vi "Get Data and Series JSON Settings.vi"(6 "Value Only":bool, 8 "error in (no error)":errorcluster, 9 "Width":u32, 10 "XY Data":variant, 11 "XYGraph in":refnum<vi>) -> (0 "error out":errorcluster, 1 "Minimums":dbl[](array[numeric]), 2 "Maximums":dbl[](array[numeric]), 3 "Series JSON":string, 4 "Plot Y Scale Index":u32[](array[numeric]), 5 "Data JSON":string)   [LabVIEW 2015, in "Front Panel Publisher.lvlib" / "Graph.lvclass"]
uses:
  Graph.lvclass
  <vilib>/Analysis/1siggen.llb/Ramp Pattern by Samples.vi
  <vilib>/gmath/NI_Gmath.lvlib
  <vilib>/Analysis/NI_AALBase.lvlib
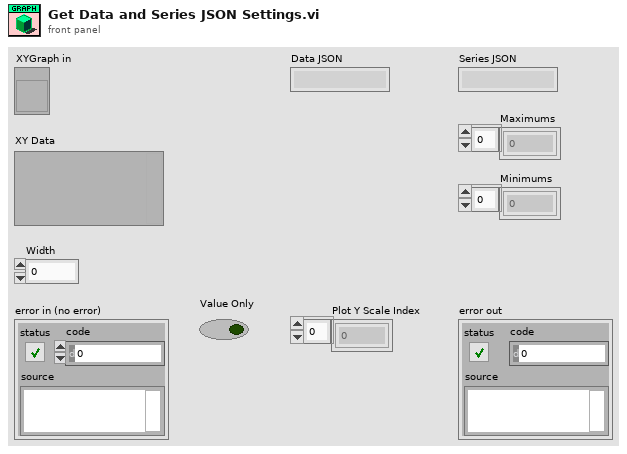
[diagram p1: front panel]
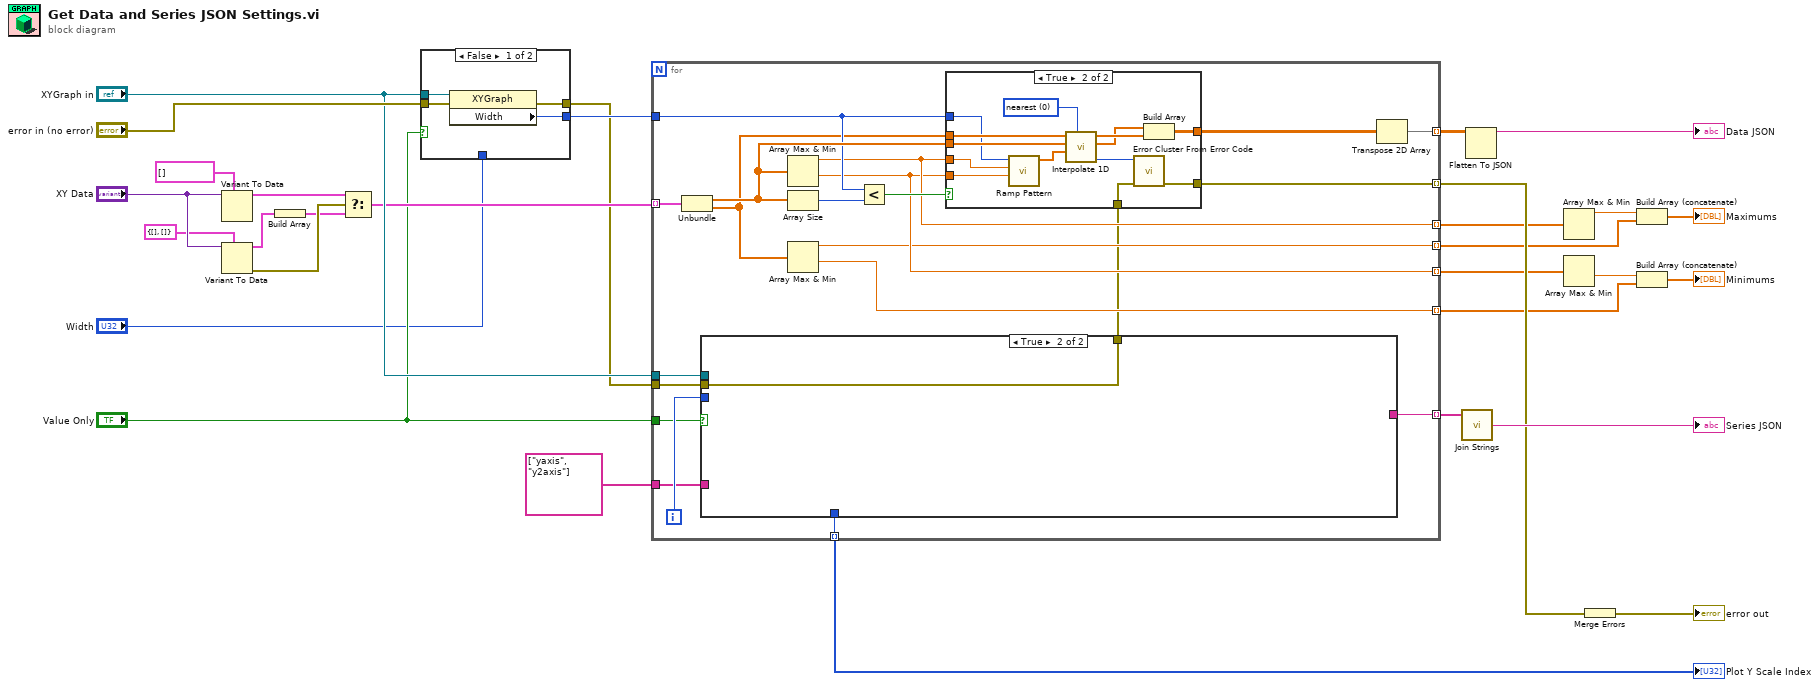
[diagram p0: block diagram]
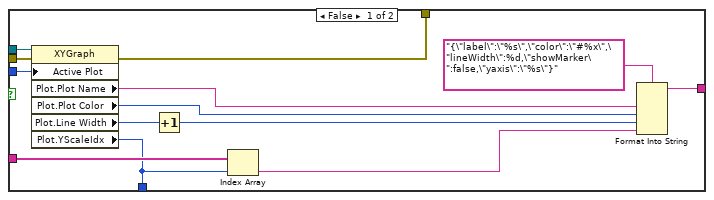
[diagram p3: hidden frame]
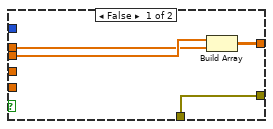
[diagram p4: hidden frame]
diagram:
  n1 = Variant To Data(type=cluster{dbl[], dbl[]}[] [], Variant="XY Data") -> (data=w15:cluster{dbl[], dbl[]}[])  [unwired: 1 in, 1 out]
  n2 = Variant To Data(type=cluster{dbl[], dbl[]} {[], []}, Variant="XY Data") -> (data=w14:cluster{dbl[], dbl[]}, error out=w16:errorcluster)  [unwired: 1 in]
  n3 = Build Array(w14) -> (w13:cluster{dbl[], dbl[]}[])
  n4 = Select(t=w15, s=w16, f=w13) -> (s? t:f=w12:cluster{dbl[], dbl[]}[])
  n5 = case shown="False" "Value Only" {
    tunnel: "error in (no error)" -> [w34 w36]
    tunnel: [w33 w35] -> w26
    tunnel: "XYGraph in" -> [w32 _]
    tunnel: [w31 w36] -> w3
    tunnel: "Width" -> [_ w35]
    frame False {
      n6 = property class="XYGraph"(reference=w32, error in=w34) -> (error out=w31:errorcluster, "Width"=w33:u32)  [unwired: 1 out]
    }
    frame True {
    }
  }
  n7 = for {
    tunnel: [w56] -> w24 mode=indexing
    tunnel: w12 -> [w54] mode=indexing
    tunnel: "XYGraph in" -> [w47]
    tunnel: [w57] -> w21 mode=indexing
    tunnel: w26 -> [w50]
    tunnel: string[] ["yaxis", "y2axis"] -> [w48]
    tunnel: [w46] -> w27 mode=indexing
    tunnel: [w45] -> w23 mode=indexing
    tunnel: [w43] -> w11 mode=indexing
    tunnel: [w42] -> w10 mode=indexing
    tunnel: [w41] -> w5 mode=indexing
    tunnel: [w40] -> w4 mode=indexing
    tunnel: w3 -> [w38]
    tunnel: "Value Only" -> [w37]
    i -> [w49]
    n8 = Unbundle(w54) -> (w52:dbl[], w44:dbl[])
    n9 = case shown="True" w37 {
      tunnel: w49 -> [w66 _]
      tunnel: w48 -> [w65 _]
      tunnel: w47 -> [w64 _]
      tunnel: [w63 _] -> w46
      tunnel: [w61 _] -> w45
      tunnel: [w59 w71] -> w39
      tunnel: w38 -> [w58 w71]
      frame False {
        n10 = property on="Property Node" class="XYGraph"(reference=w64, error in=w58, "Active Plot"=w66) -> (error out=w59:errorcluster, "Plot.Plot Name"=w68:string, "Plot.Plot Color"=w69:u32, "Plot.Line Width"=w70:u8, "Plot.YScaleIdx"=w63:u32)  [unwired: 1 out]
        n11 = Increment(x=w70) -> (x+1=w60:u8)
        n12 = Index Array(array=w65, index=w63) -> (element=w62:string)
        n13 = Format Into String(format string="{\"label\":\"%s\",\"color\":\"#%x\",\"lineWidth\":%d,\"showMarker\":false,\"yaxis\":\"%s\"}", w68, w69, w60, w62) -> (resulting string=w61:string)  [unwired: 2 in, 1 out]
      }
      frame True {
      }
    }
    n14 = Array Max & Min(array=w52) -> (max value=w43:dbl, min value=w42:dbl)  [unwired: 2 out]
    n15 = Array Size(array=w52) -> (size(s)=w51:i32)
    n16 = Array Max & Min(array=w44) -> (max value=w41:dbl, min value=w40:dbl)  [unwired: 2 out]
    n17 = Less?(x=w50, y=w51) -> (x < y?=w53:bool)
    n18 = case shown="True" w53 {
      tunnel: [w75 w88] -> w57
      tunnel: [w74 w86] -> w55
      tunnel: w44 -> [w72 w85]
      tunnel: w52 -> [w73 w79]
      tunnel: w43 -> [_ w78]
      tunnel: w42 -> [_ w77]
      tunnel: w50 -> [_ w76]
      tunnel: w39 -> [w75 w87]
      frame False {
        n19 = Build Array(w73, w72) -> (w74:dbl[][])
      }
      frame True {
        w80 = 0 items=["nearest", "linear", "spline", "cubic Hermite", "Lagrange"] ("method")
        n20 = call-poly <vilib>:"Ramp Pattern.vi"("start"=w77, "end"=w78, "samples"=w76) -> ("Ramp Pattern"=w81:dbl[])  [unwired: 7 in, 1 out]
        n21 = call <vilib>:"Interpolate 1D.vi"("method"=w80, "xi"=w81, "X"=w79, "Y"=w85) -> ("error"=w82:i32, "xi used"=w83:dbl[], "yi"=w84:dbl[])  [unwired: 5 in]
        n22 = call <vilib>:"Error Cluster From Error Code.vi"("error in (no error)"=w87, "error code (0)"=w82) -> ("error out"=w88:errorcluster)  [unwired: 7 in]
        n23 = Build Array(w83, w84) -> (w86:dbl[][])
      }
    }
    n24 = Transpose 2D Array(2D array=w55) -> (transposed array=w56:dbl[][])
  }
  "Plot Y Scale Index" <- w27
  n25 = call <vilib>:"Join Strings.vi"("Strings In"=w23) -> ("String"=→"Series JSON":string)  [unwired: 2 in]
  n26 = Flatten To JSON(anything=w24) -> (JSON string=→"Data JSON":string)  [unwired: 2 in, 1 out]
  n27 = Array Max & Min(array=w11) -> (max value=w9:dbl)  [unwired: 3 out]
  n28 = Array Max & Min(array=w10) -> (min value=w8:dbl)  [unwired: 3 out]
  n29 = Merge Errors(w21) -> (→"error out":errorcluster)
  n30 = Build Array (concatenate)(w9, w5) -> (→"Maximums":dbl[])
  n31 = Build Array (concatenate)(w8, w4) -> (→"Minimums":dbl[])
